vi "dataSampled.vi"(8 "Error In":errorcluster, 10 "Data":string, 11 "refnum in":refnum<file>) -> (0 "error out":errorcluster, 3 "refnum out":refnum<file>)   [LabVIEW 2018]
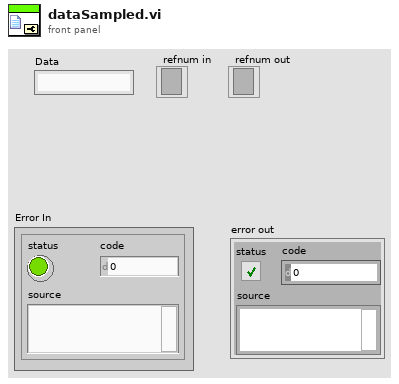
[diagram p1: front panel]
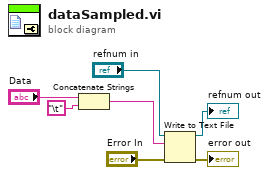
[diagram p0: block diagram]
diagram:
  n1 = Concatenate Strings("Data", "\t") -> (w2:string)
  n2 = Write to Text File(file (use dialog)="refnum in", text=w2, error in="Error In") -> (refnum out=→"refnum out":refnum<file>, error out=→"error out":errorcluster)  [unwired: 1 in, 1 out]
